vi "Init Data Object.vi"(11 "ePAS Data in":refnum<class "ePAS Data.lvclass">) -> (3 "ePAS Data out":refnum<class "ePAS Data.lvclass">)   [LabVIEW 2014, in "ePAS Data.lvclass"]
uses:
  ePAS Data.lvclass
  reusable/Data/Data.lvclass/Data.ctl
  reusable/PAS/Data/Main/PAS Data.lvclass
  reusable/Data/Data.lvclass
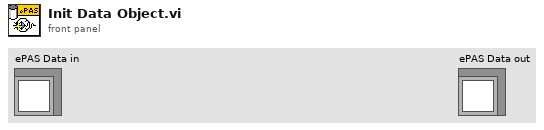
[diagram p1: front panel]
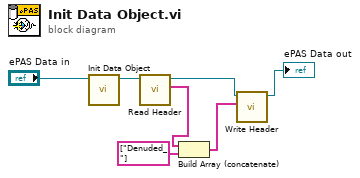
[diagram p0: block diagram]
diagram:
  n1 = call-parent "Init Data Object.vi"("Data in"="ePAS Data in") -> ("Data out"=w6:refnum<class "ePAS Data.lvclass">)  [unwired: 10 in]
  n2 = call "Read Header.vi"("Data in"=w6) -> ("Header"=w5:string[], "Data out"=w2:refnum<class "ePAS Data.lvclass">)  [unwired: 8 in, 1 out]
  n3 = Build Array (concatenate)(w5, string[] ["Denuded_"] ("element")) -> (w3:string[])
  n4 = call "Write Header.vi"("Header"=w3, "Data in"=w2) -> ("Data out"=→"ePAS Data out":refnum<class "ePAS Data.lvclass">)  [unwired: 8 in, 1 out]
